vi "OTSU.vi"() -> (0 "After OTSU":dbl[][](graph), 1 "after otsu":dbl[][](array[numeric]))   [LabVIEW 2021]
panel:
  in  "Input array":dbl[][](array[numeric])
  out "OTSU":cluster{dbl[], dbl[]}(graph)={[0.0, 1.0, 2.0, 3.0, 4.0, 5.0, 6.0, 7.0, 8.0, 9.0, 10.0, 11.0, 12.0, 13.0, 14.0, 15.0, 16.0, 17.0, 18.0, 19.0, 20.0, 21.0, 22.0, 23.0, 24.0, 25.0, 26.0, 27.0, 28.0, 29.0, 30.0, 31.0, 32.0, 33.0, 34.0, 35.0, 36.0, 37.0, 38.0, 39.0, 40.0, 41.0, 42.0, 43.0, 44.0, 45.0, 46.0, 47.0, 48.0, 49.0, 50.0, 51.0, 52.0, 53.0, 54.0, 55.0, 56.0, 57.0, 58.0, 59.0, 60.0, 61.0, 62.0, 63.0, 64.0, 65.0, 66.0, 67.0, 68.0, 69.0, 70.0, 71.0, 72.0, 73.0, 74.0, 75.0, 76.0, 77.0, 78.0, 79.0, 80.0, 81.0, 82.0, 83.0, 84.0, 85.0, 86.0, 87.0, 88.0, 89.0, 90.0, 91.0, 92.0, 93.0, 94.0, 95.0, 96.0, 97.0, 98.0, 99.0, 100.0, 101.0, 102.0, 103.0, 104.0, 105.0, 106.0, 107.0, 108.0, 109.0, 110.0, 111.0, 112.0, 113.0, 114.0, 115.0, 116.0, 117.0, 118.0, 119.0, 120.0, 121.0, 122.0, 123.0, 124.0, 125.0, 126.0, 127.0, 128.0, 129.0, 130.0, 131.0, 132.0, 133.0, 134.0, 135.0, 136.0, 137.0, 138.0, 139.0, 140.0, 141.0, 142.0, 143.0, 144.0, 145.0, 146.0, 147.0, 148.0, 149.0, 150.0, 151.0, 152.0, 153.0, 154.0, 155.0, 156.0, 157.0, 158.0, 159.0, 160.0, 161.0, 162.0, 163.0, 164.0, 165.0, 166.0, 167.0, 168.0, 169.0, 170.0, 171.0, 172.0, 173.0, 174.0, 175.0, 176.0, 177.0, 178.0, 179.0, 180.0, 181.0, 182.0, 183.0, 184.0, 185.0, 186.0, 187.0, 188.0, 189.0, 190.0, 191.0, 192.0, 193.0, 194.0, 195.0, 196.0, 197.0, 198.0, 199.0, 200.0, 201.0, 202.0, 203.0, 204.0, 205.0, 206.0, 207.0, 208.0, 209.0, 210.0, 211.0, 212.0, 213.0, 214.0, 215.0, 216.0, 217.0, 218.0, 219.0, 220.0, 221.0, 222.0, 223.0, 224.0, 225.0, 226.0, 227.0, 228.0, 229.0, 230.0, 231.0, 232.0, 233.0, 234.0, 235.0, 236.0, 237.0, 238.0, 239.0, 240.0, 241.0, 242.0, 243.0, 244.0, 245.0, 246.0, 247.0, 248.0, 249.0, 250.0, 251.0, 252.0, 253.0, 254.0], [nan, nan, nan, nan, nan, nan, nan, nan, nan, 11.798636931096558, 11.798636931096558, 11.798636931096558, 17.234659226011626, 17.234659226011626, 17.234659226011626, 18.14107883314994, 18.14107883314994, 18.14107883314994, 15.213427749130187, 15.213427749130187, 15.213427749130187, 10.77581166696673, 10.77581166696673, 10.77581166696673, 5.831771205026132, 5.831771205026132, 5.831771205026132, 2.77175702460166, 2.77175702460166, 2.77175702460166, 0.6842536363112686, 0.6842536363112686, 0.6842536363112686]}
  out "Uf":dbl=32.99999999999979
  out "Ub":dbl=14.540322580645162
  out "Wf":dbl=0.002012072434607659
  out "Wb":dbl=0.9979879275653923
  out "Intensity-pixel map":cluster{dbl[], dbl[]}(graph)={[0.0, 1.0, 2.0, 3.0, 4.0, 5.0, 6.0, 7.0, 8.0, 9.0, 10.0, 11.0, 12.0, 13.0, 14.0, 15.0, 16.0, 17.0, 18.0, 19.0, 20.0, 21.0, 22.0, 23.0, 24.0, 25.0, 26.0, 27.0, 28.0, 29.0, 30.0, 31.0, 32.0, 33.0, 34.0, 35.0, 36.0, 37.0, 38.0, 39.0, 40.0, 41.0, 42.0, 43.0, 44.0, 45.0, 46.0, 47.0, 48.0, 49.0, 50.0, 51.0, 52.0, 53.0, 54.0, 55.0, 56.0, 57.0, 58.0, 59.0, 60.0, 61.0, 62.0, 63.0, 64.0, 65.0, 66.0, 67.0, 68.0, 69.0, 70.0, 71.0, 72.0, 73.0, 74.0, 75.0, 76.0, 77.0, 78.0, 79.0, 80.0, 81.0, 82.0, 83.0, 84.0, 85.0, 86.0, 87.0, 88.0, 89.0, 90.0, 91.0, 92.0, 93.0, 94.0, 95.0, 96.0, 97.0, 98.0, 99.0, 100.0, 101.0, 102.0, 103.0, 104.0, 105.0, 106.0, 107.0, 108.0, 109.0, 110.0, 111.0, 112.0, 113.0, 114.0, 115.0, 116.0, 117.0, 118.0, 119.0, 120.0, 121.0, 122.0, 123.0, 124.0, 125.0, 126.0, 127.0, 128.0, 129.0, 130.0, 131.0, 132.0, 133.0, 134.0, 135.0, 136.0, 137.0, 138.0, 139.0, 140.0, 141.0, 142.0, 143.0, 144.0, 145.0, 146.0, 147.0, 148.0, 149.0, 150.0, 151.0, 152.0, 153.0, 154.0, 155.0, 156.0, 157.0, 158.0, 159.0, 160.0, 161.0, 162.0, 163.0, 164.0, 165.0, 166.0, 167.0, 168.0, 169.0, 170.0, 171.0, 172.0, 173.0, 174.0, 175.0, 176.0, 177.0, 178.0, 179.0, 180.0, 181.0, 182.0, 183.0, 184.0, 185.0, 186.0, 187.0, 188.0, 189.0, 190.0, 191.0, 192.0, 193.0, 194.0, 195.0, 196.0, 197.0, 198.0, 199.0, 200.0, 201.0, 202.0, 203.0, 204.0, 205.0, 206.0, 207.0, 208.0, 209.0, 210.0, 211.0, 212.0, 213.0, 214.0, 215.0, 216.0, 217.0, 218.0, 219.0, 220.0, 221.0, 222.0, 223.0, 224.0, 225.0, 226.0, 227.0, 228.0, 229.0, 230.0, 231.0, 232.0, 233.0, 234.0, 235.0, 236.0, 237.0, 238.0, 239.0, 240.0, 241.0, 242.0, 243.0, 244.0, 245.0, 246.0, 247.0, 248.0, 249.0, 250.0, 251.0, 252.0, 253.0, 254.0], [0.0, 0.0, 0.0, 0.0, 0.0, 0.0, 0.0, 0.0, 0.0, 410.0, 0.0, 0.0, 313.0, 0.0, 0.0, 284.0, 0.0, 0.0, 231.0, 0.0, 0.0, 131.0, 0.0, 0.0, 77.0, 0.0, 0.0, 29.0, 0.0, 0.0, 13.0, 0.0, 0.0, 3.0, 0.0, 0.0, 0.0, 0.0, 0.0, 0.0, 0.0, 0.0, 0.0, 0.0, 0.0, 0.0, 0.0, 0.0, 0.0, 0.0, 0.0, 0.0, 0.0, 0.0, 0.0, 0.0, 0.0, 0.0, 0.0, 0.0, 0.0, 0.0, 0.0, 0.0, 0.0, 0.0, 0.0, 0.0, 0.0, 0.0, 0.0, 0.0, 0.0, 0.0, 0.0, 0.0, 0.0, 0.0, 0.0, 0.0, 0.0, 0.0, 0.0, 0.0, 0.0, 0.0, 0.0, 0.0, 0.0, 0.0, 0.0, 0.0, 0.0, 0.0, 0.0, 0.0, 0.0, 0.0, 0.0, 0.0, 0.0, 0.0, 0.0, 0.0, 0.0, 0.0, 0.0, 0.0, 0.0, 0.0, 0.0, 0.0, 0.0, 0.0, 0.0, 0.0, 0.0, 0.0, 0.0, 0.0, 0.0, 0.0, 0.0, 0.0, 0.0, 0.0, 0.0, 0.0, 0.0, 0.0, 0.0, 0.0, 0.0, 0.0, 0.0, 0.0, 0.0, 0.0, 0.0, 0.0, 0.0, 0.0, 0.0, 0.0, 0.0, 0.0, 0.0, 0.0, 0.0, 0.0, 0.0, 0.0, 0.0, 0.0, 0.0, 0.0, 0.0, 0.0, 0.0, 0.0, 0.0, 0.0, 0.0, 0.0, 0.0, 0.0, 0.0, 0.0, 0.0, 0.0, 0.0, 0.0, 0.0, 0.0, 0.0, 0.0, 0.0, 0.0, 0.0, 0.0, 0.0, 0.0, 0.0, 0.0, 0.0, 0.0, 0.0, 0.0, 0.0, 0.0, 0.0, 0.0, 0.0, 0.0, 0.0, 0.0, 0.0, 0.0, 0.0, 0.0, 0.0, 0.0, 0.0, 0.0, 0.0, 0.0, 0.0, 0.0, 0.0, 0.0, 0.0, 0.0, 0.0, 0.0, 0.0, 0.0, 0.0, 0.0, 0.0, 0.0, 0.0, 0.0, 0.0, 0.0, 0.0, 0.0, 0.0, 0.0, 0.0, 0.0, 0.0, 0.0, 0.0, 0.0, 0.0, 0.0, 0.0, 0.0, 0.0, 0.0, 0.0, 0.0, 0.0, 0.0, 0.0, 0.0, 0.0, 0.0, 0.0, 0.0, 0.0, 0.0, 0.0, 0.0, 0.0]}
  out "min":dbl
  out "max":dbl=33.0
  out "input":dbl[][](graph)
  # "大津算法"
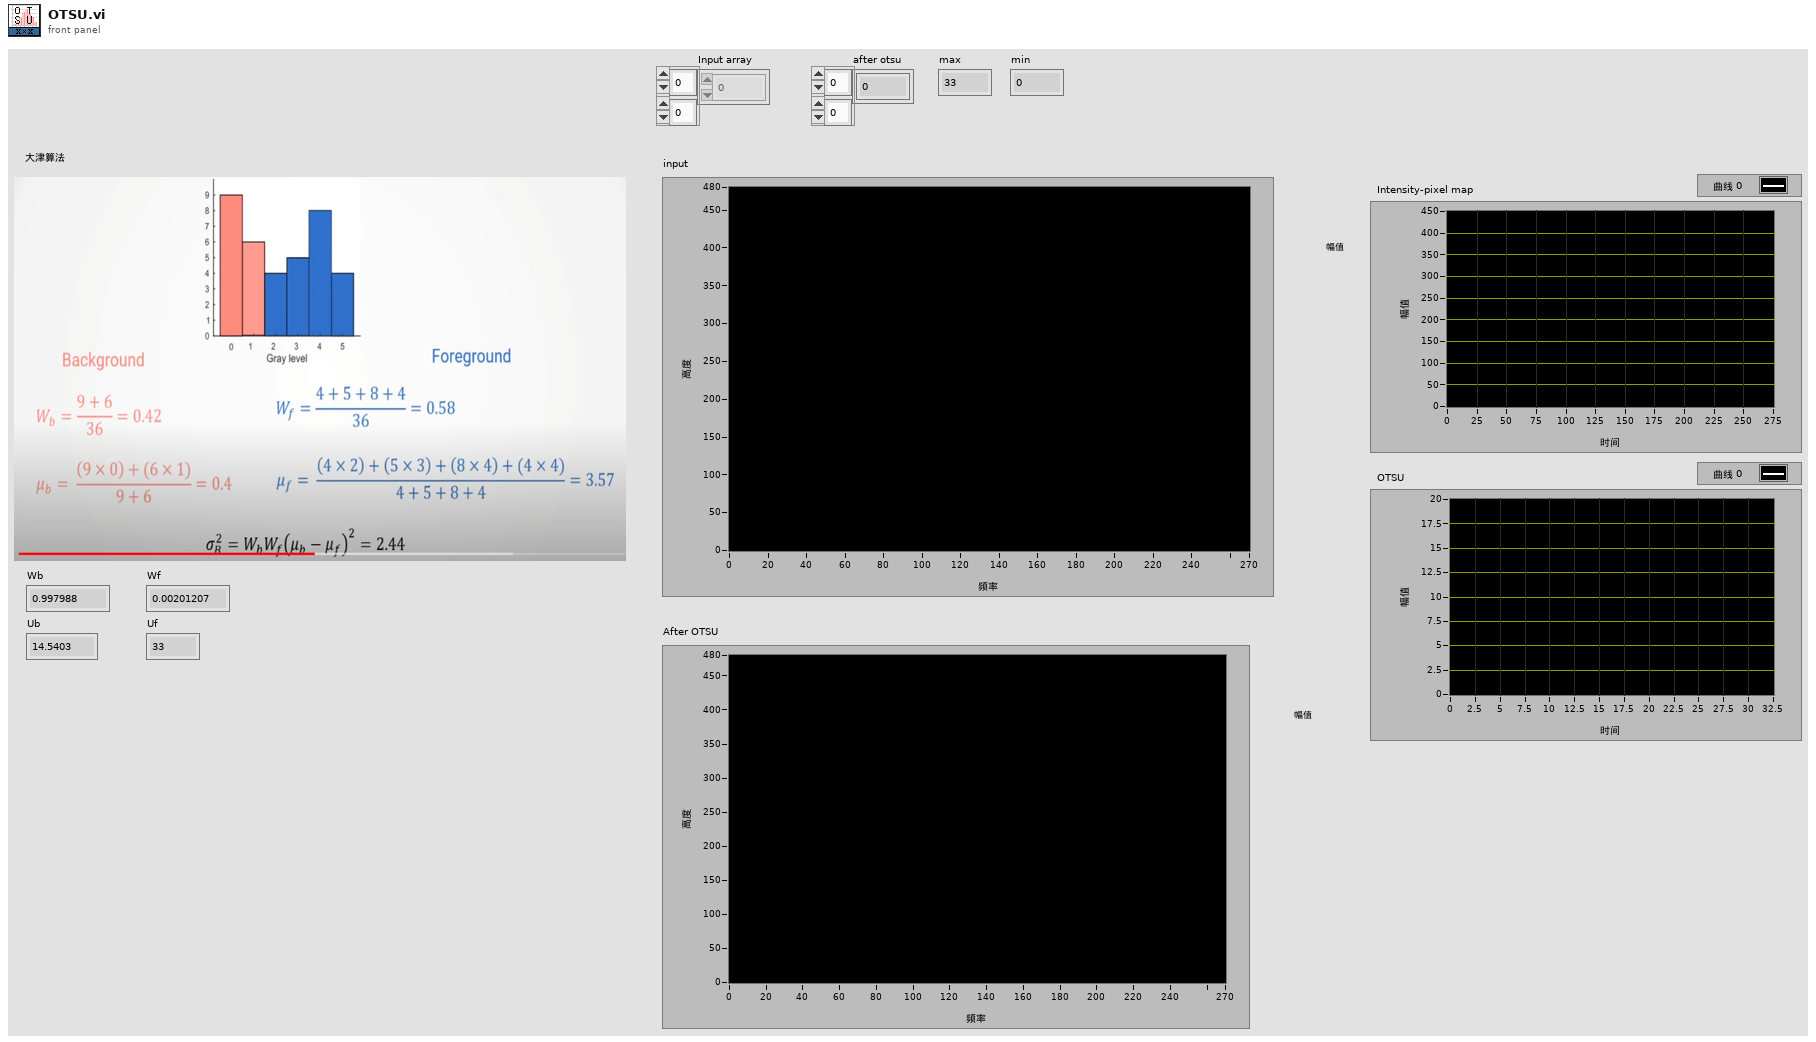
[diagram p1: front panel]
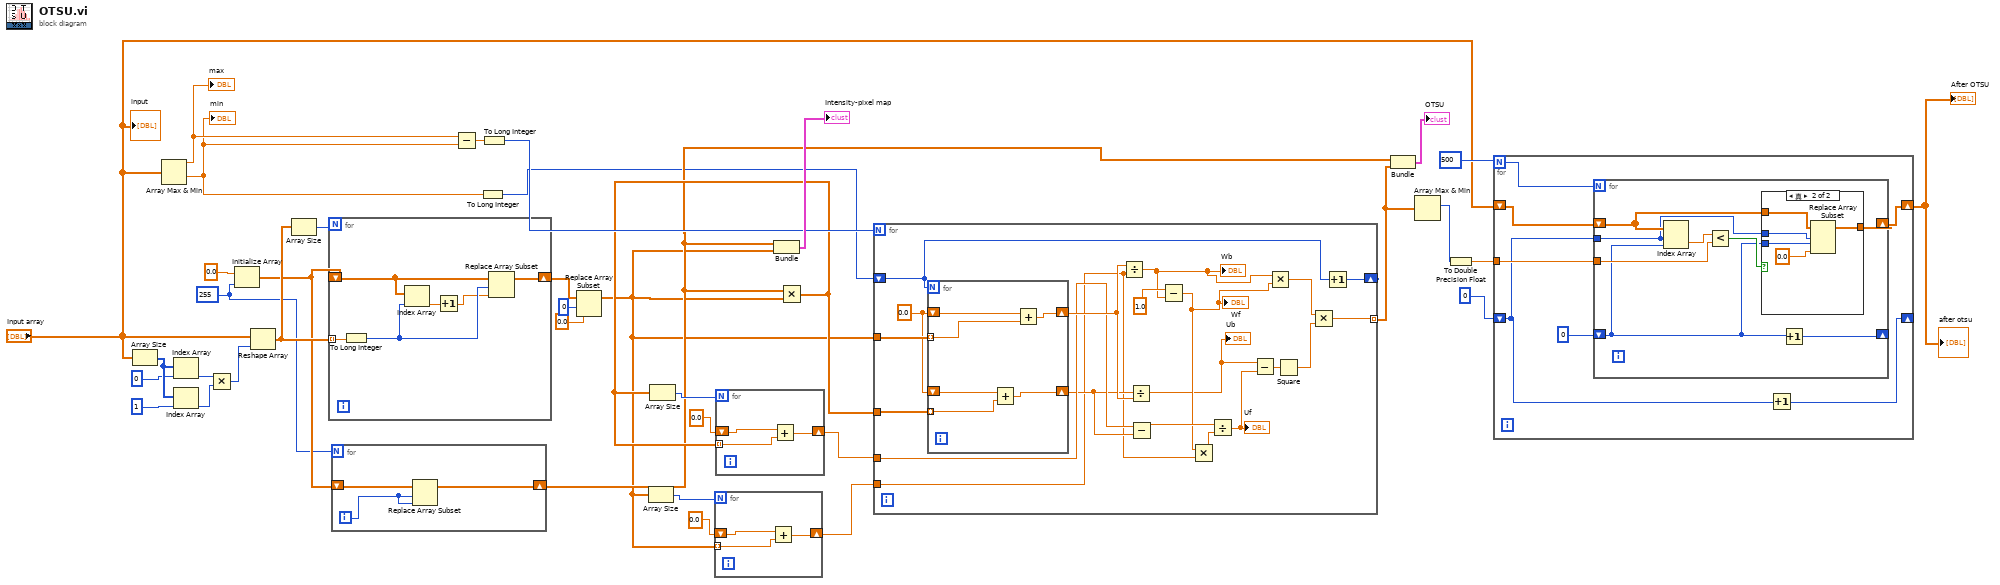
[diagram p0: block diagram]
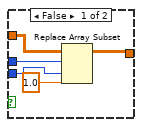
[diagram p2: hidden frame]
diagram:
  w24 = 255 ("维数大小")
  n1 = Array Size(array="Input array") -> (size(s)=w37:i32[])
  n2 = Array Max & Min(array="Input array") -> (max value=w23:dbl, min value=w20:dbl)  [unwired: 2 out]
  "max" <- w23
  "min" <- w20
  n3 = Index Array(array=w37, index=0 ("索引")) -> (element=w34:i32)
  n4 = Index Array(array=w37, index=1 ("索引")) -> (element=w33:i32)
  n5 = Multiply(x=w34, y=w33) -> (x*y=w32:i32)
  n6 = Initialize Array(0.0 ("元素"), w24) -> (w27:dbl[])
  n7 = Reshape Array("Input array", w32) -> (w29:dbl[])
  n8 = Array Size(array=w29) -> (size(s)=w31:i32)
  n9 = for {
    N: w31 -> [_]
    shift-right: [w38] -> w11
    shift-left: w27 -> [w42]
    tunnel: w29 -> [w43] mode=indexing
    n10 = To Long Integer(number=w43) -> (32bit integer=w41:i32)
    n11 = Index Array(array=w42, index=w41) -> (element=w40:dbl)
    n12 = Increment(x=w40) -> (x+1=w39:dbl)
    n13 = Replace Array Subset(array=w42, new element=w39, index=w41) -> (w38:dbl[])
  }
  n14 = for {
    N: w24 -> [_]
    shift-right: [w45] -> w14
    shift-left: w27 -> [w46]
    i -> [w44]
    n15 = Replace Array Subset(array=w46, new element=w44, index=w44) -> (w45:dbl[])
  }
  n16 = Subtract(x=w23, y=w20) -> (x-y=w26:dbl)
  n17 = To Long Integer(number=w20) -> (32bit integer=w1:i32)
  n18 = To Long Integer(number=w26) -> (32bit integer=w25:i32)
  n19 = Replace Array Subset(array=w11, new element=0.0 ("新元素/子数组"), index=0 ("索引")) -> (w10:dbl[])
  n20 = Array Size(array=w10) -> (size(s)=w19:i32)
  n21 = for {
    N: w19 -> [_]
    tunnel: w10 -> [w48] mode=indexing
    shift-right: [w47] -> w21
    shift-left: 0.0 -> [w49]
    n22 = Add(x=w49, y=w48) -> (x+y=w47:dbl)
  }
  n23 = Bundle(w14, w10) -> (→"Intensity-pixel map":cluster{dbl[], dbl[]})  [unwired: 1 in]
  n24 = Multiply(x=w14, y=w10) -> (x*y=w16:dbl[])
  n25 = Array Size(array=w16) -> (size(s)=w17:i32)
  n26 = for {
    N: w17 -> [_]
    tunnel: w16 -> [w51] mode=indexing
    shift-right: [w50] -> w15
    shift-left: 0.0 -> [w52]
    n27 = Add(x=w52, y=w51) -> (x+y=w50:dbl)
  }
  n28 = for {
    N: w25 -> [_]
    tunnel: w21 -> [w64]
    tunnel: w10 -> [w72]
    tunnel: w16 -> [w70]
    tunnel: w15 -> [w67]
    tunnel: [w55] -> w8 mode=indexing
    shift-right: [w54] -> _
    shift-left: w1 -> [w53]
    w69 = 0.0 ("元素")
    n29 = for {
      N: w53 -> [_]
      shift-right: [w77] -> w68
      shift-left: w69 -> [w78]
      tunnel: w72 -> [w76] mode=indexing
      tunnel: w70 -> [w74] mode=indexing
      shift-right: [w73] -> w66
      shift-left: w69 -> [w75]
      n30 = Add(x=w75, y=w74) -> (x+y=w73:dbl)
      n31 = Add(x=w78, y=w76) -> (x+y=w77:dbl)
    }
    n32 = Divide(x=w68, y=w64) -> (x/y=w62:dbl)
    "Wb" <- w62
    n33 = Divide(x=w66, y=w68) -> (x/y=w60:dbl)
    "Ub" <- w60
    n34 = Subtract(x=w67, y=w66) -> (x-y=w65:dbl)
    n35 = Subtract(x=1.0 ("元素"), y=w62) -> (x-y=w61:dbl)
    "Wf" <- w61
    n36 = Multiply(x=w61, y=w64) -> (x*y=w63:dbl)
    n37 = Divide(x=w65, y=w63) -> (x/y=w59:dbl)
    "Uf" <- w59
    n38 = Subtract(x=w60, y=w59) -> (x-y=w58:dbl)
    n39 = Multiply(x=w62, y=w61) -> (x*y=w57:dbl)
    n40 = Square(x=w58) -> (x^2=w56:dbl)
    n41 = Multiply(x=w57, y=w56) -> (x*y=w55:dbl)
    n42 = Increment(x=w53) -> (x+1=w54:i32)
  }
  n43 = Bundle(w14, w8) -> (→"OTSU":cluster{dbl[], dbl[]})  [unwired: 1 in]
  n44 = Array Max & Min(array=w8) -> (max index (indices)=w6:i32)  [unwired: 3 out]
  n45 = To Double Precision Float(number=w6) -> (double precision float=w5:dbl)
  n46 = for {
    N: 500 -> [w85]
    shift-right: [w82] -> w3
    shift-left: "Input array" -> [w83]
    tunnel: w5 -> [w84]
    shift-right: [w79] -> _
    shift-left: 0 -> [w80]
    n47 = for {
      N: w85 -> [_]
      shift-right: [w92] -> w82
      shift-left: w83 -> [w91]
      tunnel: w84 -> [w93]
      shift-right: [w88] -> _
      shift-left: 0 -> [w87]
      tunnel: w80 -> [w86]
      n48 = Index Array(array=w91, index (row)=w86, index (col)=w87) -> (element=w90:dbl)
      n49 = Less?(x=w90, y=w93) -> (x < y?=w89:bool)
      n50 = case shown="真" w89 {
        tunnel: w91 -> [w98 w103]
        tunnel: [w97 w102] -> w92
        tunnel: w87 -> [w95 w100]
        tunnel: w86 -> [w96 w99]
        frame False {
          n51 = Replace Array Subset(array=w98, new element=1.0 ("新元素/子数组"), index (row)=w96, index (col)=w95) -> (w97:dbl[][])
        }
        frame True {
          n52 = Replace Array Subset(array=w103, new element=0.0 ("新元素/子数组"), index (row)=w99, index (col)=w100) -> (w102:dbl[][])
        }
      }
      n53 = Increment(x=w87) -> (x+1=w88:i32)
    }
    n54 = Increment(x=w80) -> (x+1=w79:i32)
  }
  "After OTSU" <- w3
  "after otsu" <- w3
  "input" <- "Input array"
